vi "3D-十字标 -正面.vi"(4 "Color":u32(colorbox)=16711680, 6 "error in (no error)":errorcluster, 8 "radius":dbl, 10 "Target Point":cluster{"X":dbl, "Y":dbl}, 11 "输入图片":T1(plugin-control)) -> (0 "error out":errorcluster, 3 "输出图片":T1(plugin-control))   [LabVIEW 2017]
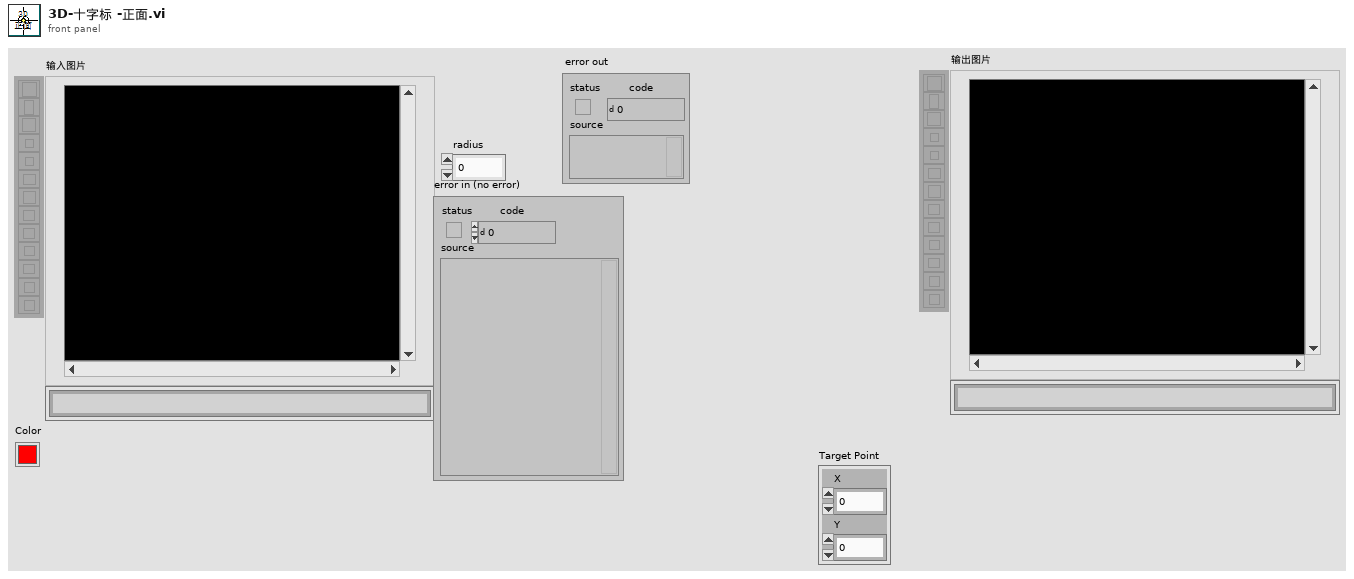
[diagram p1: front panel]
types:
  T1 = typedef "IMAQ Image.ctl" = refnum<image>
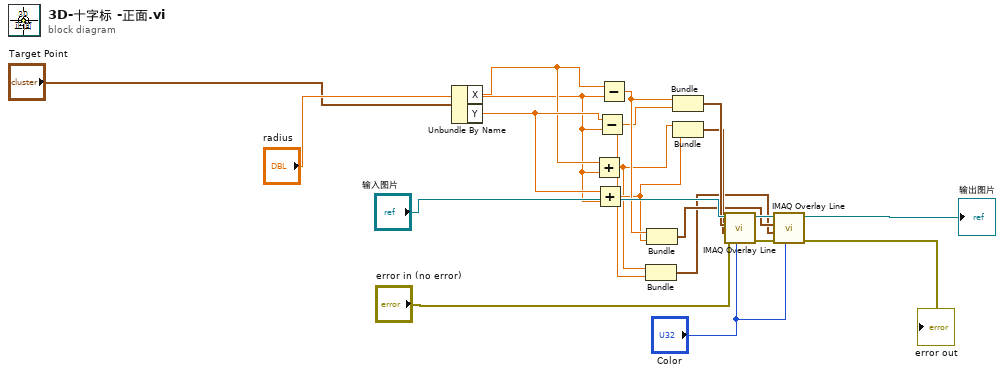
[diagram p0: block diagram]
diagram:
  n1 = Unbundle By Name("Target Point") -> ("X"=w11:dbl, "Y"=w12:dbl)
  n2 = Add(x=w11, y="radius") -> (x+y=w5:dbl)
  n3 = Add(x=w12, y="radius") -> (x+y=w7:dbl)
  n4 = Subtract(x=w12, y="radius") -> (x-y=w4:dbl)
  n5 = Subtract(x=w11, y="radius") -> (x-y=w8:dbl)
  n6 = Bundle(w5, w4) -> (w3:cluster{dbl, dbl})  [unwired: 1 in]
  n7 = Bundle(w8, w7) -> (w6:cluster{dbl, dbl})  [unwired: 1 in]
  n8 = Bundle(w8, w4) -> (w13:cluster{dbl, dbl})  [unwired: 1 in]
  n9 = Bundle(w5, w7) -> (w9:cluster{dbl, dbl})  [unwired: 1 in]
  n10 = call "IMAQ Overlay Line"("Color"="Color", "error in (no error)"="error in (no error)", "End Point"=w9, "Start Point"=w13, "Image"="输入图片") -> ("error out"=w17:errorcluster, "Image Out"=w19:T1)  [unwired: 5 in]
  n11 = call "IMAQ Overlay Line"("Color"="Color", "error in (no error)"=w17, "End Point"=w3, "Start Point"=w6, "Image"=w19) -> ("error out"=→"error out":errorcluster, "Image Out"=→"输出图片":T1)  [unwired: 5 in]
